vi "comms_BT_Read_Packet.vi"(8 "error in":errorcluster, 11 "connection ID":refnum<k31>) -> (0 "error out":errorcluster, 2 "Data Out":string, 3 "connection ID out":refnum<k31>)   [LabVIEW 2016]
panel:
  in  "Bytes in Packet":i32=394
  in  "Size offset":i32=1
  out "Surplus":string
  out "BT Sync?":bool
  in  "Pkt Offset":i32=6
  # "s"
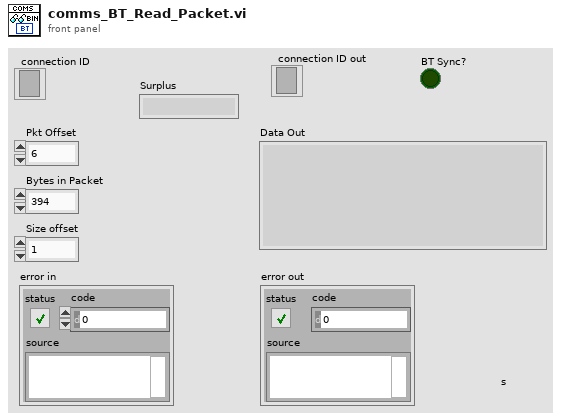
[diagram p1: front panel]
types:
  T1 = enum16{"Standard", "Buffered", "CRLF", "Immediate"}
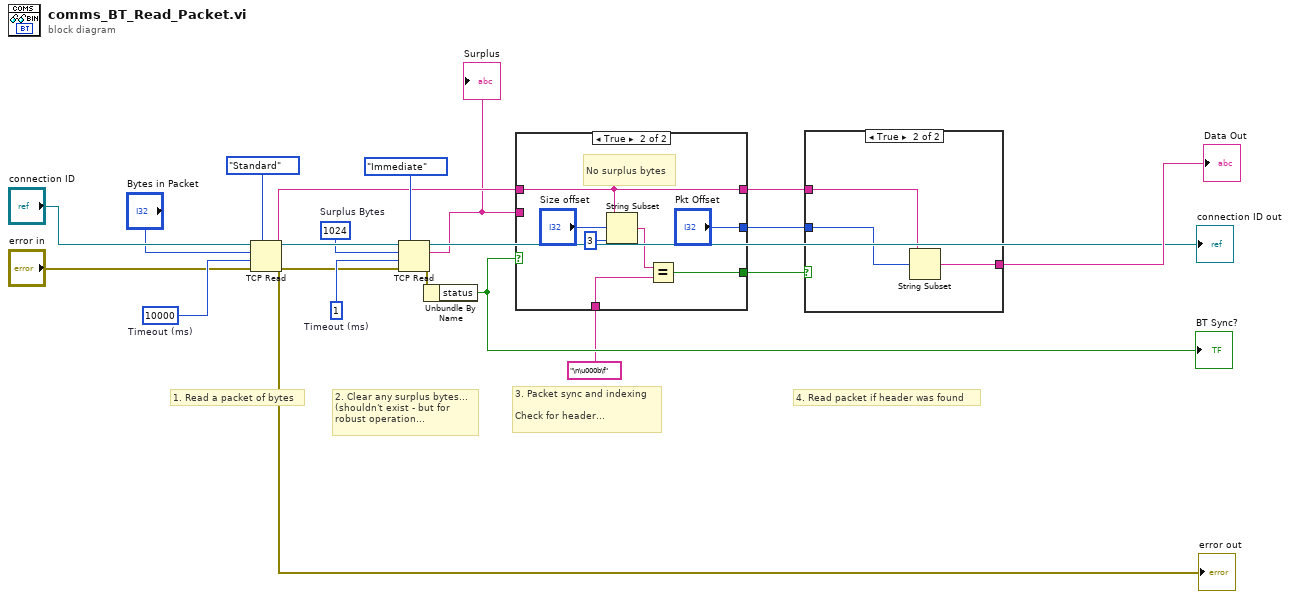
[diagram p0: block diagram]
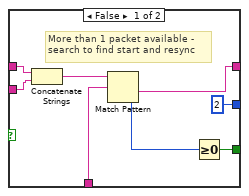
[diagram p2: hidden frame]
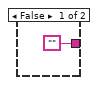
[diagram p3: hidden frame]
diagram:
  w10 = 1  # Timeout (ms)
  w11 = 1024  # Surplus Bytes
  w16 = 10000  # Timeout (ms)
  # "3. Packet sync and indexing\n\nCheck for header..."
  # "2. Clear any surplus bytes...\n(shouldn't exist - but for \nrobust operation..."
  # "1. Read a packet of bytes"
  # "4. Read packet if header was found"
  n1 = TCP Read(connection ID="connection ID", bytes to read="Bytes in Packet", error in (no error)="error in", 7:T1."Standard" ("mode (standard)"), 9:w16) -> (connection ID out=w14:refnum<k31>, data out=w6:string, error out=w9:errorcluster)
  "error out" <- w9
  n2 = TCP Read(connection ID=w14, bytes to read=w11, error in (no error)=w9, 7:T1."Immediate" ("mode (standard)"), 9:w10) -> (connection ID out=→"connection ID out":refnum<k31>, data out=w5:string, error out=w8:errorcluster)
  "Surplus" <- w5
  n3 = Unbundle By Name(w8) -> ("status"=w7:bool)
  "BT Sync?" <- w7
  n4 = case shown="True" w7 {
    tunnel: w6 -> [w28 w31]
    tunnel: [w25 w31] -> w2
    tunnel: w5 -> [w27 _]
    tunnel: "\n\u000b\f" ("y") -> [w23 w32]
    tunnel: [w22 w30] -> w3
    tunnel: [2 ("Pkt Offset") "Pkt Offset"] -> w1
    frame False {
      # "More than 1 packet available - \nsearch to find start and resync"
      n5 = Concatenate Strings(w28, w27) -> (w26:string)
      n6 = Match Pattern(string=w26, regular expression=w23) -> (after substring=w25:string, offset past match=w21:i32)  [unwired: 1 in, 2 out]
      n7 = Greater Or Equal To 0?(x=w21) -> (x >= 0?=w22:bool)
    }
    frame True {
      # "No surplus bytes"
      n8 = String Subset(string=w31, offset (0)="Size offset", length (rest)=3 ("length (rest)")) -> (substring=w34:string)
      n9 = Equal?(x=w34, y=w32) -> (x = y?=w30:bool)
    }
  }
  n10 = case shown="True" w3 {
    tunnel: ["" w39] -> w20
    tunnel: w2 -> [_ w38]
    tunnel: w1 -> [_ w37]
    frame False {
    }
    frame True {
      n11 = String Subset(string=w38, offset (0)=w37) -> (substring=w39:string)  [unwired: 1 in]
    }
  }
  "Data Out" <- w20
